vi "TMCM351- resolution.vi"(4 "错误输入":errorcluster caption="错误输入（无错误）", 5 "reasulotion":T1(ring), 6 "motor":u8(ring) items=["x", "y", "z"], 7 "com in":refnum<visa-resource-name>) -> (0 "错误输出":errorcluster, 3 "com out":refnum<visa-resource-name>)   [LabVIEW 2018]
uses:
  module_param.vi
panel:
  # "设置分辨率"
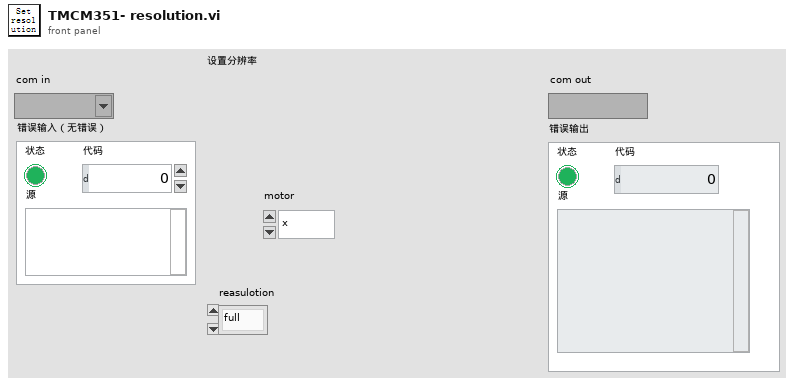
[diagram p1: front panel]
types:
  T1 = enum8{"full", "half", "4", "8", "16", "32", "64"}
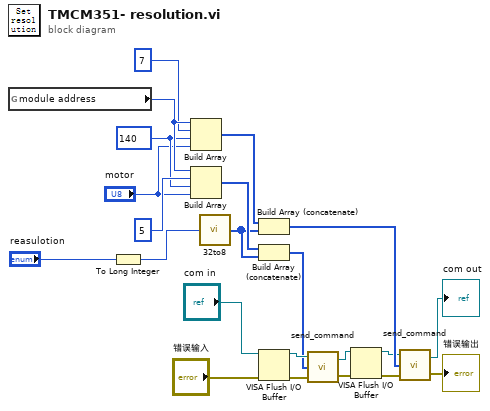
[diagram p0: block diagram]
diagram:
  w11 = u8 140
  n1 = global read "module_param.vi" "module address"() -> (w13:u8)
  n2 = To Long Integer(number="reasulotion") -> (32bit integer=w14:i32)
  n3 = Build Array(w13, u8 7 ("元素"), w11, "motor") -> (w9:u8[])
  n4 = Build Array(w13, u8 5, w11, "motor") -> (w17:u8[])
  n5 = call "32to8.vi"("32data_in"=w14) -> ("8Array"=w8:u8[])
  n6 = Build Array (concatenate)(w9, w8) -> (w7:u8[])
  n7 = Build Array (concatenate)(w17, w8) -> (w16:u8[])
  n8 = VISA Flush I/O Buffer(VISA resource name="com in", error in (no error)="错误输入") -> (VISA resource name out=w19:refnum<visa-resource-name>, error out=w18:errorcluster)  [unwired: 1 in]
  n9 = call "send_command.vi"("错误输入"=w18, 3:w16, "com in"=w19) -> ("错误输出"=w5:errorcluster, "com out"=w6:refnum<visa-resource-name>)
  n10 = VISA Flush I/O Buffer(VISA resource name=w6, error in (no error)=w5) -> (VISA resource name out=w4:refnum<visa-resource-name>, error out=w3:errorcluster)  [unwired: 1 in]
  n11 = call "send_command.vi"("错误输入"=w3, 3:w7, "com in"=w4) -> ("错误输出"=→"错误输出":errorcluster, "com out"=→"com out":refnum<visa-resource-name>)
